vi "test sender-receiver.vi"() -> ()   [LabVIEW 2019]
panel:
  in  "kruispunt":string
  out "bericht":string
  in  "STOP":bool
  in  "START":bool
  in  "stop 2":bool
  out "address":u32
  out "port":u16
  in  "stop":bool
  in  "vooruit":bool
  in  "achteruit":bool
  in  "links":bool
  in  "rechts":bool
  in  "linksvooruit":bool
  in  "rechtsvooruit":bool
  in  "rechtsachter":bool
  in  "linksachter":bool
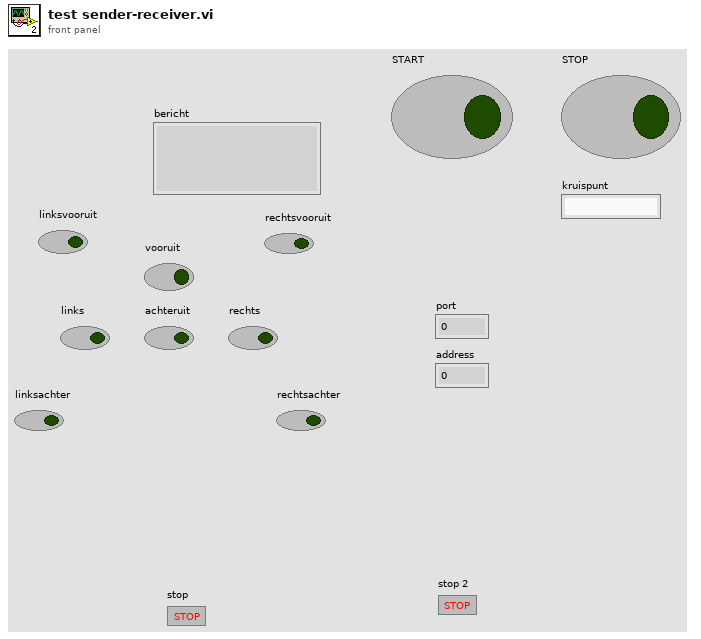
[diagram p1: front panel]
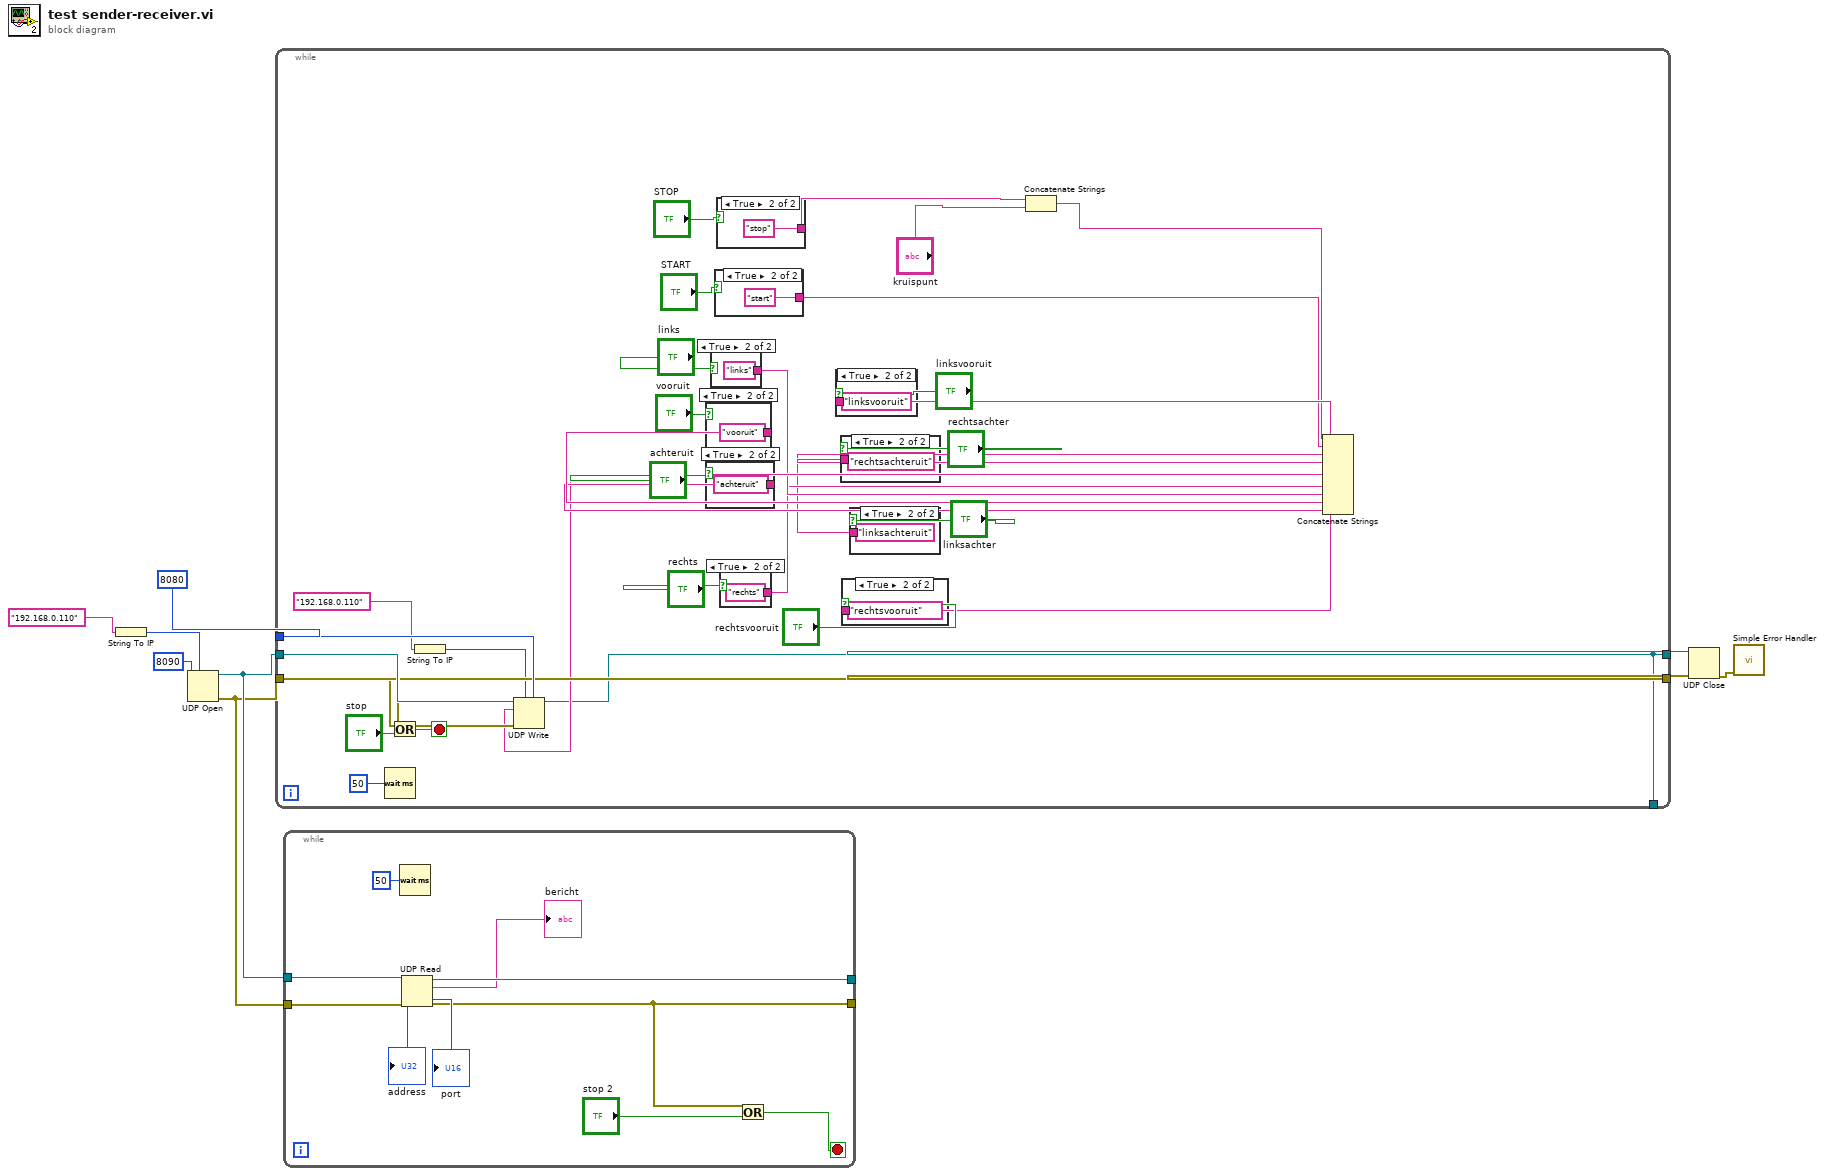
[diagram p0: block diagram]
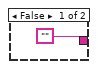
[diagram p2: hidden frame]
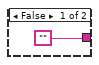
[diagram p3: hidden frame]
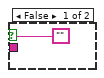
[diagram p4: hidden frame]
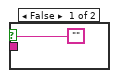
[diagram p5: hidden frame]
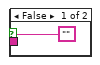
[diagram p6: hidden frame]
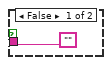
[diagram p7: hidden frame]
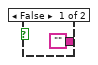
[diagram p8: hidden frame]
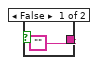
[diagram p9: hidden frame]
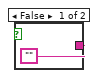
[diagram p10: hidden frame]
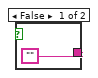
[diagram p11: hidden frame]
diagram:
  n1 = String To IP(1:"192.168.0.110") -> (0:w4:u32)
  n2 = UDP Open(7:w4, 11:8090) -> (port=w3:refnum<k16>, 0:w2:errorcluster)  [unwired: 3 in, 1 out]
  n3 = while {
    tunnel: w3 -> [w42]
    tunnel: w2 -> [w41]
    tunnel: 8080 -> [w37]
    tunnel: [w18] -> w1
    tunnel: [w36] -> w7
    tunnel: [w18] -> _
    stop <- w39 stop-if-true
    n4 = Wait (ms)(milliseconds to wait=50) -> ()  [unwired: 1 out]
    n5 = String To IP(1:"192.168.0.110") -> (0:w29:u32)
    n6 = case shown="True" "vooruit" {
      tunnel: ["" "vooruit"] -> w33
      frame False {
      }
      frame True {
      }
    }
    n7 = case shown="True" "achteruit" {
      tunnel: ["" "achteruit"] -> w32
      frame False {
      }
      frame True {
      }
    }
    n8 = case shown="True" "links" {
      tunnel: ["" "links"] -> w28
      frame False {
      }
      frame True {
      }
    }
    n9 = case shown="True" "START" {
      tunnel: ["" "start"] -> w15
      frame False {
      }
      frame True {
      }
    }
    n10 = case shown="True" "STOP" {
      tunnel: ["" "stop"] -> w11
      frame False {
      }
      frame True {
      }
    }
    n11 = case shown="True" "rechts" {
      tunnel: ["" "rechts"] -> w26
      frame False {
      }
      frame True {
      }
    }
    n12 = case shown="True" "linksvooruit" {
      tunnel: ["" "linksvooruit"] -> w22
      frame False {
      }
      frame True {
      }
    }
    n13 = case shown="True" "rechtsachter" {
      tunnel: ["" "rechtsachteruit"] -> w20
      frame False {
      }
      frame True {
      }
    }
    n14 = case shown="True" "rechtsvooruit" {
      tunnel: ["" "rechtsvooruit"] -> w23
      frame False {
      }
      frame True {
      }
    }
    n15 = case shown="True" "linksachter" {
      tunnel: ["" "linksachteruit"] -> w19
      frame False {
      }
      frame True {
      }
    }
    n16 = Concatenate Strings(w11, "kruispunt") -> (w12:string)
    n17 = Concatenate Strings(w12, w15, w19, w20, w22, w23, w26, w28, w33, w32) -> (w31:string)
    n18 = UDP Write(address=w29, port or service name=w37, connection ID=w42, data in=w31, 8:w41) -> (error out=w36:errorcluster, 3:w18:refnum<k16>)  [unwired: 1 in]
    n19 = Or(x=w36, y="stop") -> (x .or. y?=w39:bool)
  }
  n20 = while {
    tunnel: w3 -> [w72]
    tunnel: w2 -> [w71]
    tunnel: [w68] -> _
    tunnel: [w67] -> _
    stop <- w65 stop-if-true
    n21 = Wait (ms)(milliseconds to wait=u32 50) -> ()  [unwired: 1 out]
    n22 = UDP Read(connection ID=w72, 8:w71) -> (data out=→"bericht":string, error out=w67:errorcluster, 3:w68:refnum<k16>, 4:→"port":u16, 6:→"address":u32)  [unwired: 2 in]
    n23 = Or(x=w67, y="stop 2") -> (x .or. y?=w65:bool)
  }
  n24 = UDP Close(connection ID=w1, 8:w7) -> (error out=w6:errorcluster)  [unwired: 1 out]
  n25 = call <vilib>:"Simple Error Handler.vi"("error in (no error)"=w6) -> ()  [unwired: 4 in, 5 out]
